vi "ItemSelection_ItemIDToRef.vi"(8 "error in (no error)":errorcluster, 10 "Item":T1) -> (0 "error out":errorcluster, 2 "Item Refnum":refnum<vi>)   [LabVIEW 2014, in "ItemSelection.lvlib"]
uses:
  ItemSelection.lvlib
  <resource>/Framework/Providers/API/ItemRef.ctl
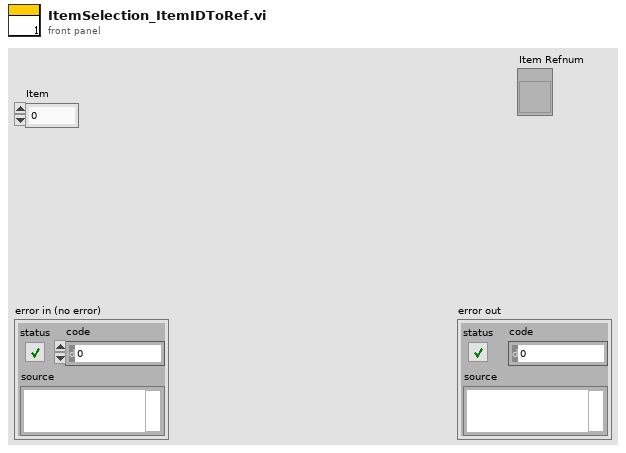
[diagram p1: front panel]
types:
  T1 = typedef "ItemRef.ctl" = u64
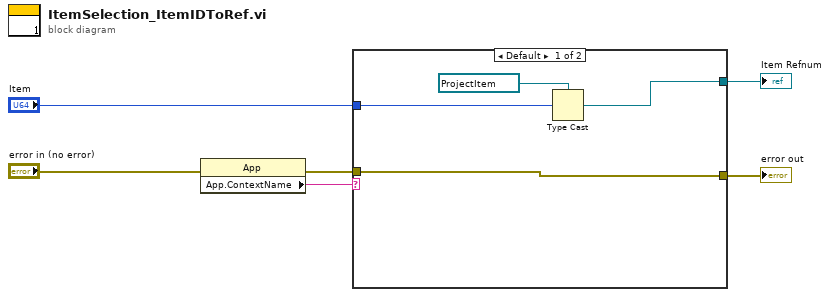
[diagram p0: block diagram]
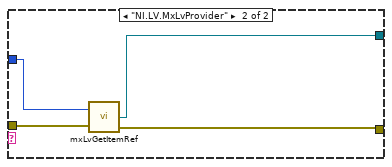
[diagram p2: hidden frame]
diagram:
  n1 = property class="App"(error in="error in (no error)") -> (error out=w5:errorcluster, "App.ContextName"=w6:string)  [unwired: 1 in, 1 out]
  n2 = case shown="Default" w6 {
    tunnel: w5 -> [w10 w14]
    tunnel: [w10 w11] -> w3
    tunnel: "Item" -> [w8 w12]
    tunnel: [w7 w13] -> w1
    frame Default {
      n3 = Type Cast(type=refnum<vi> refnum ("Item Refnum"), x=w8) -> (*(type *) &x=w7:refnum<vi>)
    }
    frame "NI.LV.MxLvProvider" {
      n4 = call <resource>:"mxLvGetItemRef.vi"("Item"=w12, "error in"=w14) -> ("Item Refnum"=w13:refnum<vi>, "error out"=w11:errorcluster)  [unwired: 1 out]
    }
  }
  "error out" <- w3
  "Item Refnum" <- w1
